vi "KepcoDCPwr Query Current Limit.vi"(0 "VISA Session":refnum<visa-resource-name>, 5 "Model In":string, 7 "channel name (\"\")":string="\"\"", 9 "Level":bool, 11 "error in (no error)":errorcluster {"code" format="%.0x"}) -> (4 "VISA Session Out":refnum<visa-resource-name>, 6 "Model Out":string, 8 "channel name out (\"\")":string="\"\"" caption="channel name Out (\"\")", 10 "current limit":dbl format="%^.2e", 15 "error out":errorcluster {"code" format="%.0x"})   [LabVIEW 2020]
doc: "This VI returns the maximum programmable current limit that the power supply accepts for a particular voltage level on a channel for the output range to which the power supply is currently configured.\n\nLevel -Max (T), Min (F)"
uses:
  Match Regular Expression.xnode
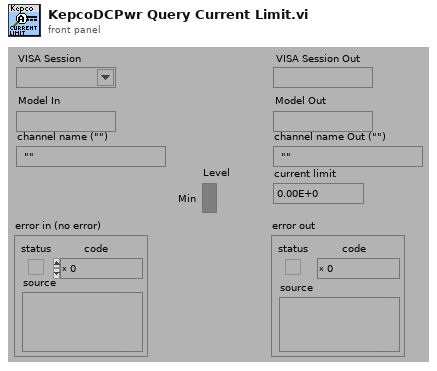
[diagram p1: front panel]
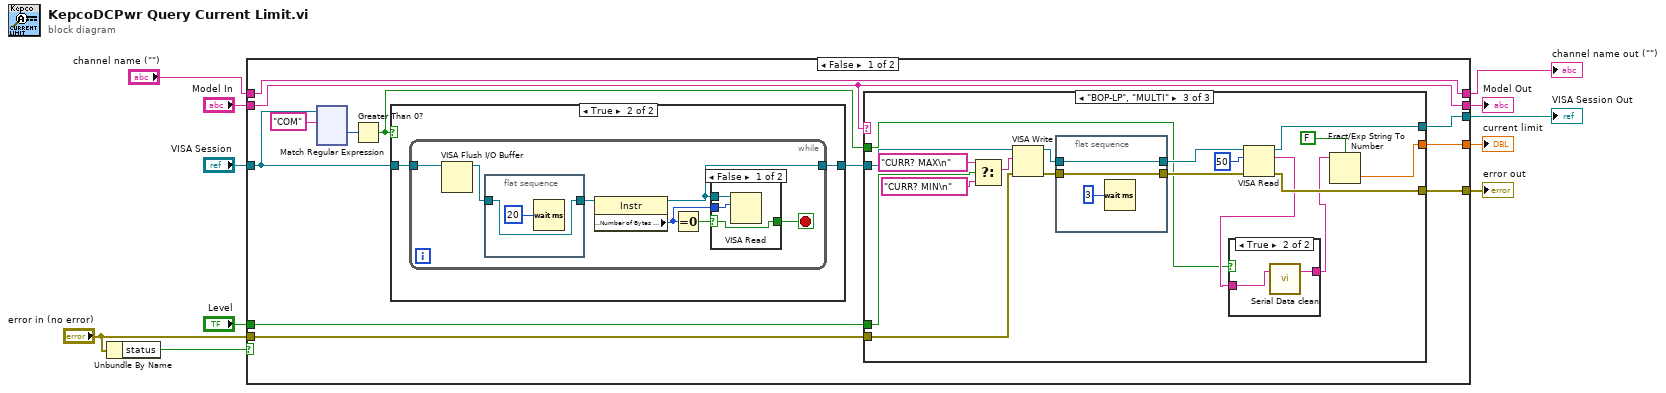
[diagram p0: block diagram]
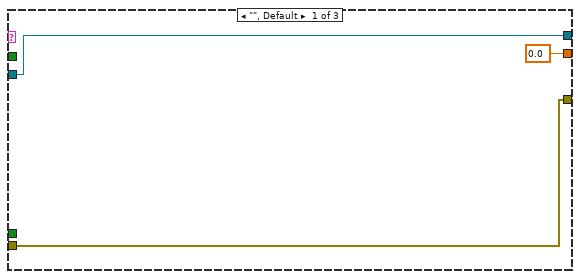
[diagram p4: hidden frame]
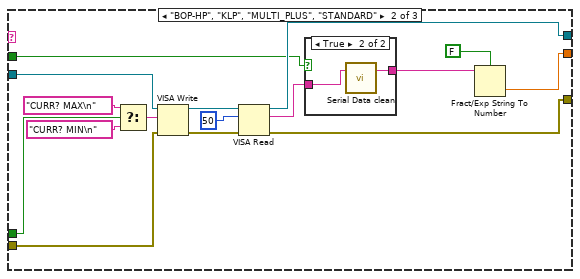
[diagram p5: hidden frame]
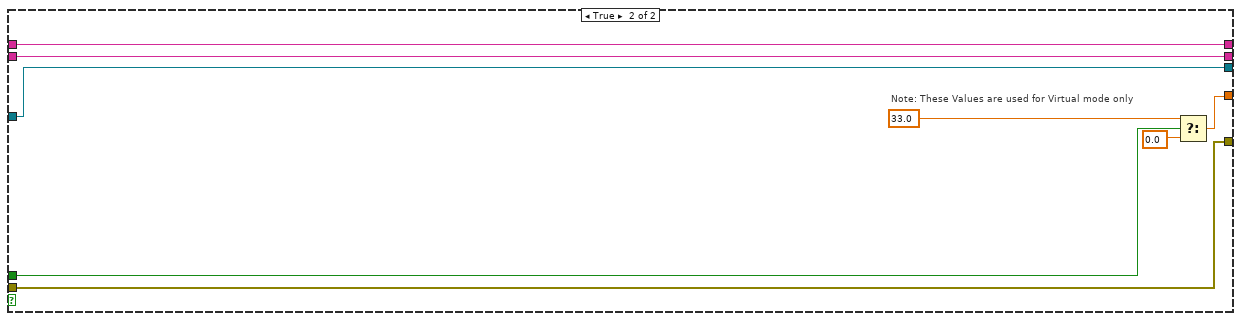
[diagram p8: hidden frame]
diagram:
  n1 = Unbundle By Name("error in (no error)") -> ("status"=w10:bool)
  n2 = case shown="False" w10 {
    tunnel: [w20 w204] -> w11
    tunnel: "error in (no error)" -> [w19 w204]
    tunnel: [w21 w203] -> w5
    tunnel: "VISA Session" -> [w13 w203]
    tunnel: [w22 w202] -> w4
    tunnel: "Model In" -> [w22 w202]
    tunnel: [w23 w201] -> w3
    tunnel: "channel name (\"\")" -> [w23 w201]
    tunnel: [w18 w199] -> w2
    tunnel: "Level" -> [w17 w200]
    frame False {
      n3 = xnode "Match Regular Expression"("input string"=w13, "regular expression"="COM") -> ("offset past match"=w15:i32)  [unwired: 2 in, 6 out]
      n4 = Greater Than 0?(x=w15) -> (x > 0?=w12:bool)
      n5 = case shown="True" w12 {
        tunnel: w13 -> [w24 w26]
        tunnel: [w24 w25] -> w14
        frame False {
        }
        frame True {
          n6 = while {
            tunnel: w26 -> [w29]
            tunnel: [w31] -> w25
            stop <- w32 stop-if-true
            n7 = VISA Flush I/O Buffer(VISA resource name=w29) -> (VISA resource name out=w28:refnum<visa-resource-name>)  [unwired: 2 in, 1 out]
            n8 = flat-sequence {
              tunnel: w28 -> [w34]
              tunnel: [w34] -> w27
              frame #0 {
                n9 = Wait (ms)(milliseconds to wait=u32 20) -> ()  [unwired: 1 out]
              }
            }
            n10 = property class="Instr"(reference=w27) -> (reference out=w31:refnum<visa-resource-name>, "Serial Settings:Number of Bytes at Serial Port"=w30:u32)  [unwired: 1 in, 1 out]
            n11 = Equal To 0?(x=w30) -> (x = 0?=w33:bool)
            n12 = case shown="False" w33 {
              selector: w33 -> [w38 w39]
              tunnel: [w38 w39] -> w32
              tunnel: w31 -> [w37 _]
              tunnel: w30 -> [w36 _]
              frame False {
                n13 = VISA Read(VISA resource name=w37, byte count=w36) -> ()  [unwired: 1 in, 4 out]
              }
              frame True {
              }
            }
          }
        }
      }
      n14 = case shown="\"BOP-LP\", \"MULTI\"" w22 {
        tunnel: w19 -> [w153 w169 w190]
        tunnel: w14 -> [w151 w168 w189]
        tunnel: [w153 w165 w188] -> w20
        tunnel: [w151 w164 w187] -> w21
        tunnel: [0.0 w162 w185] -> w18
        tunnel: w17 -> [_ w158 w181]
        tunnel: w12 -> [_ w154 w173]
        frame "", Default {
        }
        frame "BOP-HP", "KLP", "MULTI_PLUS", "STANDARD" {
          n15 = Select(t="CURR? MAX\n", s=w158, f="CURR? MIN\n") -> (s? t:f=w159:string)
          n16 = VISA Write(VISA resource name=w168, write buffer=w159, error in (no error)=w169) -> (VISA resource name out=w167:refnum<visa-resource-name>, error out=w166:errorcluster)  [unwired: 1 out]
          n17 = VISA Read(VISA resource name=w167, byte count=u32 50 ("byte count (0)"), error in (no error)=w166) -> (VISA resource name out=w164:refnum<visa-resource-name>, read buffer=w156:string, error out=w165:errorcluster)  [unwired: 1 out]
          n18 = case shown="True" w154 {
            tunnel: [w170 w171] -> w155
            tunnel: w156 -> [w170 w172]
            frame False {
            }
            frame True {
              n19 = call "Serial Data clean.vi"("string"=w172) -> ("Stripped of Xon Xoff"=w171:string)  [unwired: 2 in]
            }
          }
          n20 = Fract/Exp String To Number(use system decimal point (T)=FALSE, string=w155) -> (number=w162:dbl)  [unwired: 2 in, 1 out]
        }
        frame "BOP-LP", "MULTI" {
          n21 = Select(t="CURR? MAX\n", s=w181, f="CURR? MIN\n") -> (s? t:f=w182:string)
          n22 = VISA Write(VISA resource name=w189, write buffer=w182, error in (no error)=w190) -> (VISA resource name out=w180:refnum<visa-resource-name>, error out=w178:errorcluster)  [unwired: 1 out]
          n23 = flat-sequence {
            tunnel: [w196] -> w179
            tunnel: w180 -> [w196]
            tunnel: w178 -> [w195]
            tunnel: [w195] -> w177
            frame #0 {
              n24 = Wait (ms)(milliseconds to wait=u32 3 ("byte count (0)")) -> ()  [unwired: 1 out]
            }
          }
          n25 = VISA Read(VISA resource name=w179, byte count=u32 50 ("byte count (0)"), error in (no error)=w177) -> (VISA resource name out=w187:refnum<visa-resource-name>, read buffer=w175:string, error out=w188:errorcluster)  [unwired: 1 out]
          n26 = case shown="True" w173 {
            tunnel: [w191 w192] -> w174
            tunnel: w175 -> [w191 w193]
            frame False {
            }
            frame True {
              n27 = call "Serial Data clean.vi"("string"=w193) -> ("Stripped of Xon Xoff"=w192:string)  [unwired: 2 in]
            }
          }
          n28 = Fract/Exp String To Number(use system decimal point (T)=FALSE, string=w174) -> (number=w185:dbl)  [unwired: 2 in, 1 out]
        }
      }
    }
    frame True {
      # "Note: These Values are used for Virtual mode only"
      n29 = Select(t=33.0, s=w200, f=0.0) -> (s? t:f=w199:dbl)
    }
  }
  "error out" <- w11
  "channel name out (\"\")" <- w3
  "Model Out" <- w4
  "VISA Session Out" <- w5
  "current limit" <- w2
